vi "K to C.vi"(11 "Temperature (K)":dbl) -> (3 "Temperature (C)":dbl)   [LabVIEW 2019]
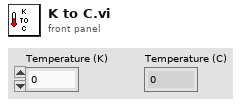
[diagram p1: front panel]
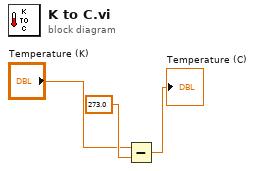
[diagram p0: block diagram]
diagram:
  n1 = Subtract(x="Temperature (K)", y=273.0) -> (x-y=→"Temperature (C)":dbl)
